vi "AFG3352X.ProcCases.vi"(0 "i ref in":refnum<vi>, 1 "selector":string, 2 "Data":T1, 3 "call cluster":T2={"Object"="", "Selector"="", "CallType"=enum."synchronous", "Async Object"="", "Async Selector"="", "Data Descriptor"="", "Data"=[], "Error #"=0, "Expire"=0}, 5 "error in (no error)":errorcluster) -> (14 "i ref out":refnum<vi>, 17 "answer cluster":T2={"Object"="", "Selector"="", "CallType"=enum."synchronous", "Async Object"="", "Async Selector"="", "Data Descriptor"="", "Data"=[], "Error #"=0, "Expire"=0}, 19 "error out":errorcluster)   [LabVIEW 2014, in "AFG3352X.lvlib"]
doc: "This method is called by a process from within the default case in the event loop. The methods of a class that are linked to events will be called from THIS method. Add your code here."
uses:
  AFG3352X.lvlib
  CS_Core/CSSystem/CoreDefs/CoreDefs.call_type.ctl
  CS_Core/BaseProcess/BaseProcess.descriptor string definition.ctl
  CS_Core/CSSystem/CoreDefs/CoreDefs.rawDataType.ctl
  CS_Core/CSSystem/CoreLib/CoreLib.string 2 byte array.vi
  CS_Core/CSSystem/CoreLib/CoreLib.byte array 2 short.vi
  CS_Core/CSSystem/CoreLib/CoreLib.byte array 2 string.vi
  CS_Core/CSSystem/CoreLib/CoreLib.byte array 2 short array.vi
  CS_Core/CSSystem/CoreLib/CoreLib.byte array 2 int.vi
  CS_Core/CSSystem/CoreLib/CoreLib.byte array 2 double.vi
  CS_Core/CSSystem/CoreLib/CoreLib.byte array 2 double array.vi
  CS_Core/CSSystem/CoreLib/CoreLib.lvlib
  CS_Core/BaseProcess/BaseProcess.lvlib
  CS_Core/CSApplicationBaseClasses/AFGBase/AFGBase.lvlib
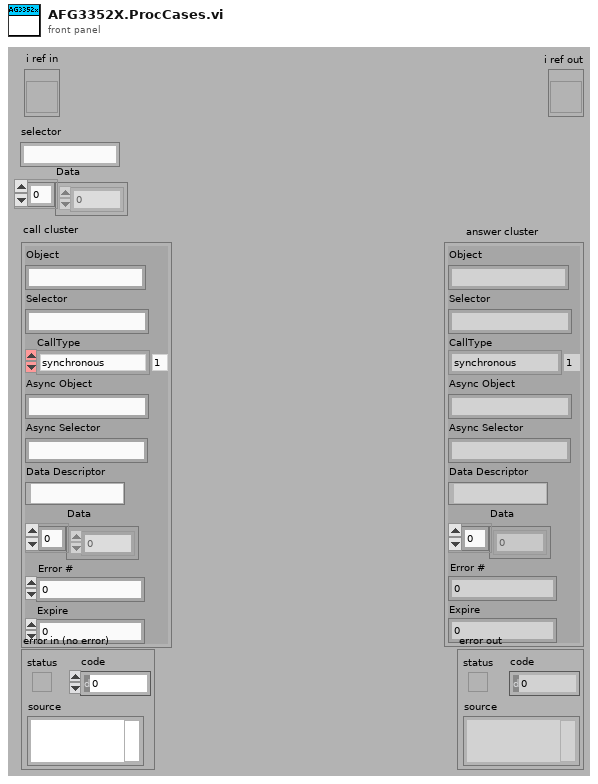
[diagram p1: front panel]
types:
  T1 = typedef "CoreDefs.rawDataType.ctl" = i8[]
  T2 = typedef "CoreDefs.call_type.ctl" = cluster{"Object":string, "Selector":string, "CallType":enum16{"simple", "synchronous", "asynchronous"}, "Async Object":string, "Async Selector":string, "Data Descriptor":T3, "Data":T1, "Error #":i32, "Expire":u32}
  T3 = typedef "BaseProcess.lvlib/BaseProcess.descriptor string definition.ctl" = string
  T4 = typedef "AFG3352X.lvlib/AFG3352X.i attribute.ctl" = cluster{"Act2ndValues":cluster{"frequency":dbl, "amplitude":dbl, "phase":dbl, "DCOffset":dbl, "waveformType":T5, "enableOutput":bool, "trigger":i16[], "serviceIDs":cluster{"frequencyID":i32, "amplitudeID":i32, "phaseID":i32, "DCOffsetID":i32, "waveformTypeID":i32, "enableOutputID":i32, "triggerID":i32}, "waveform":cluster{"data":waveform(dbl), "gain":dbl, "offset":dbl, "repetitionRate":dbl, "sampleRate":dbl}}, "Nom2ndValues":cluster{"frequency":dbl, "amplitude":dbl, "phase":dbl, "DCOffset":dbl, "waveformType":T5, "enableOutput":bool, "trigger":i16[], "serviceIDs":cluster{"frequencyID":i32, "amplitudeID":i32, "phaseID":i32, "DCOffsetID":i32, "waveformTypeID":i32, "enableOutputID":i32, "triggerID":i32}, "waveform":cluster{"data":waveform(dbl), "gain":dbl, "offset":dbl, "repetitionRate":dbl, "sampleRate":dbl}}, "DefaultChannel":i32, "ActAddValues":cluster{"Mode1":u16, "serviceIDs":cluster{"Mode1ID":i32, "Mode2ID":i32, "Burst1ID":i32, "Burst2ID":i32}, "Mode2":u16, "Burst1":i32, "Burst2":i32}, "NomAddValues":cluster{"Mode1":u16, "serviceIDs":cluster{"Mode1ID":i32, "Mode2ID":i32, "Burst1ID":i32, "Burst2ID":i32}, "Mode2 2":u16, "Burst1":i32, "Burst2":i32}, "enableBurstMode":bool}
  T5 = typedef "AFGBase.lvlib/AFGBase.waveformType.ctl" = enum16{"sine", "square", "ramp", "pulse", "noise", "DC", "arbitrary", "triangle", "ramp_up", "ramp_down", "amplitude modulation"}
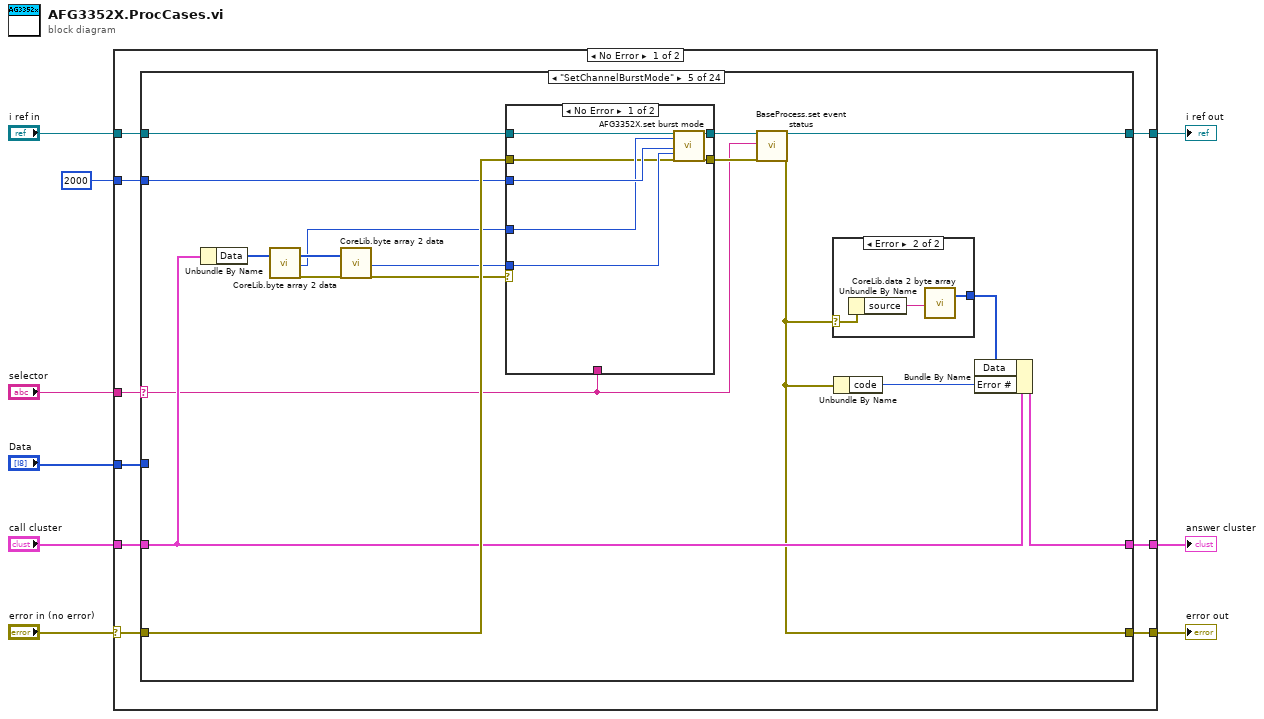
[diagram p0: block diagram]
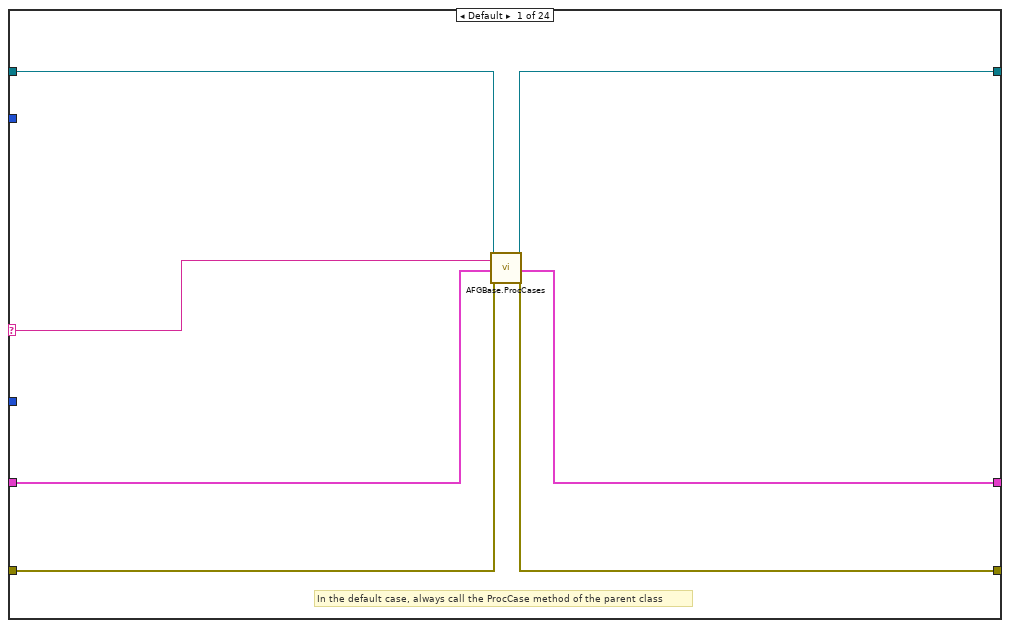
[diagram p2: hidden frame]
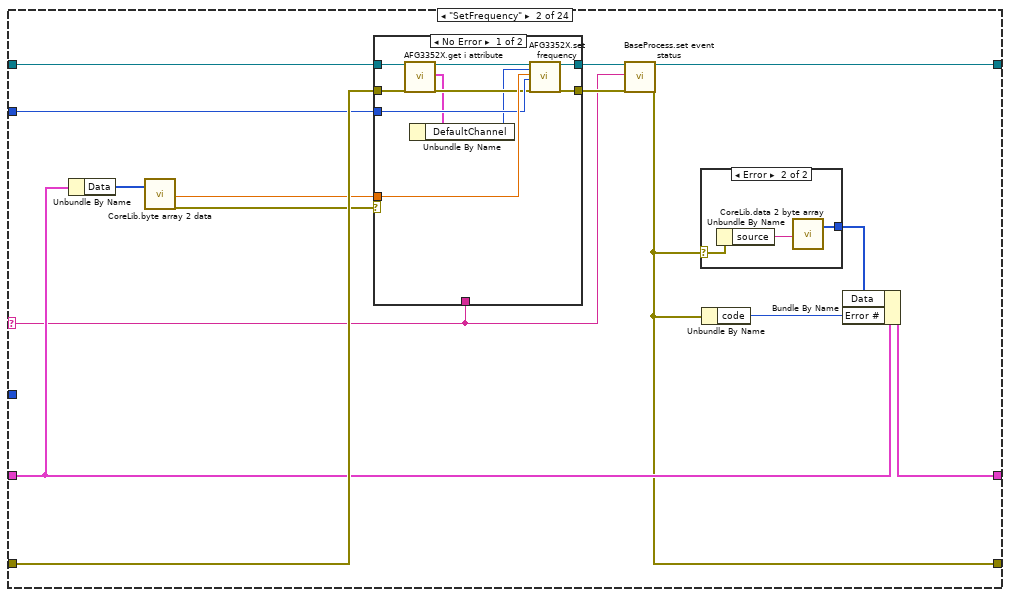
[diagram p3: hidden frame]
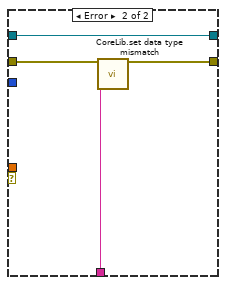
[diagram p5: hidden frame]
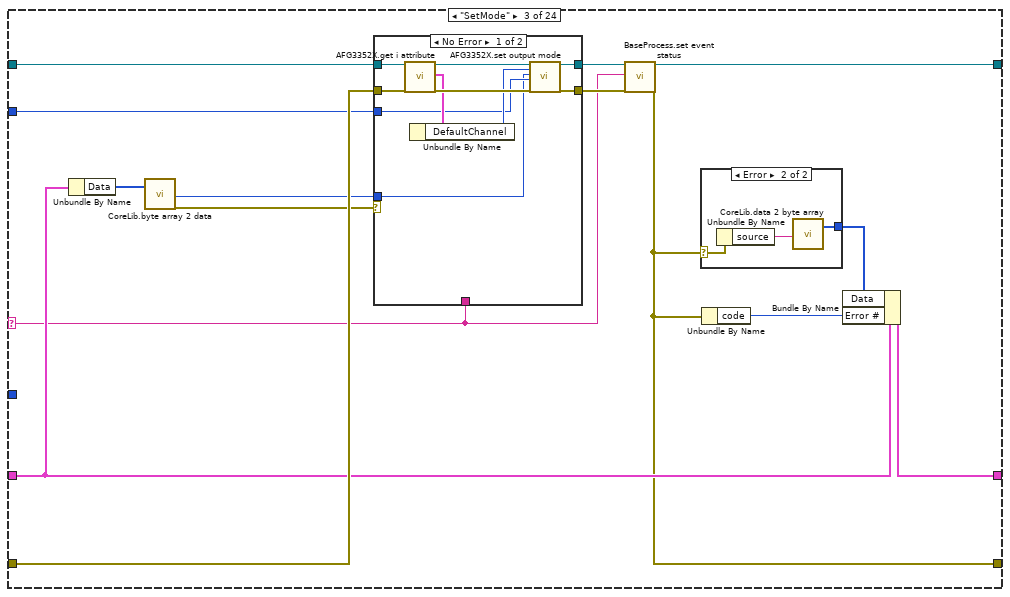
[diagram p6: hidden frame]
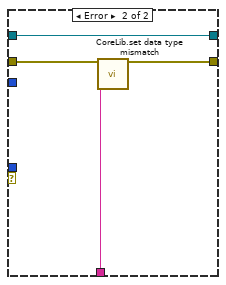
[diagram p8: hidden frame]
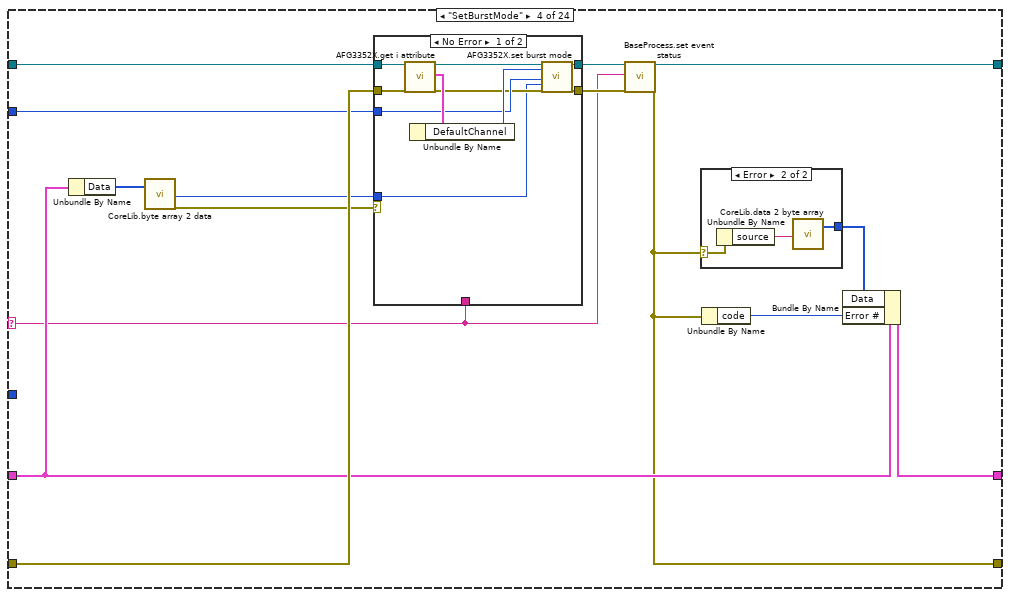
[diagram p9: hidden frame]
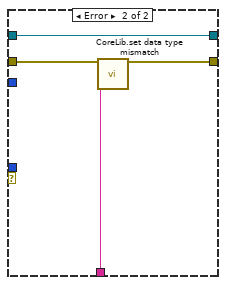
[diagram p11: hidden frame]
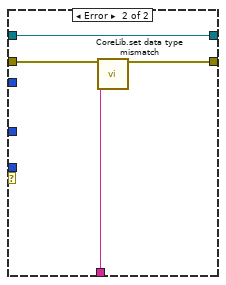
[diagram p13: hidden frame]
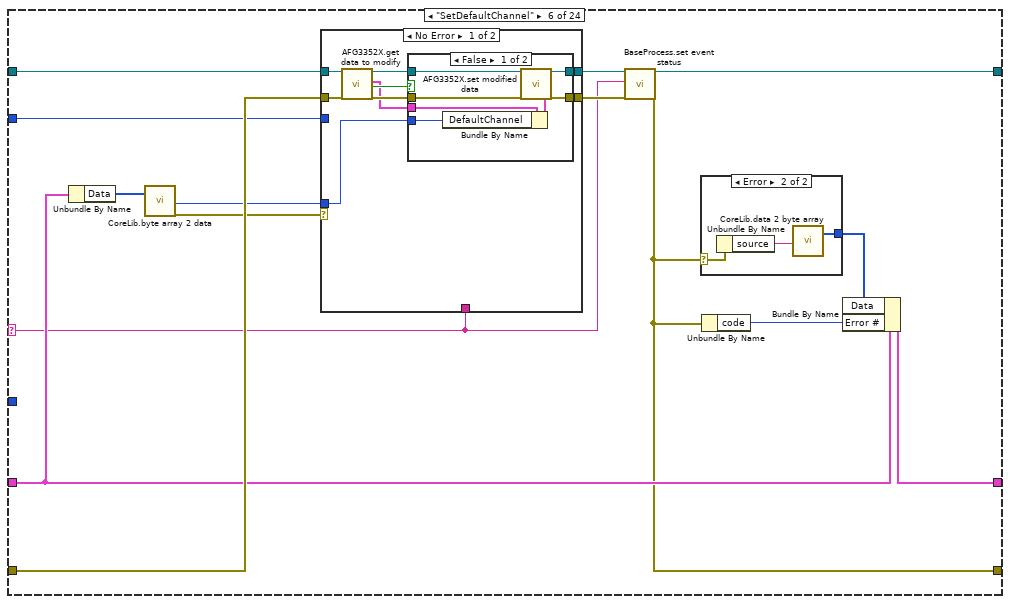
[diagram p14: hidden frame]
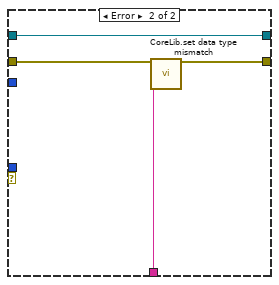
[diagram p17: hidden frame]
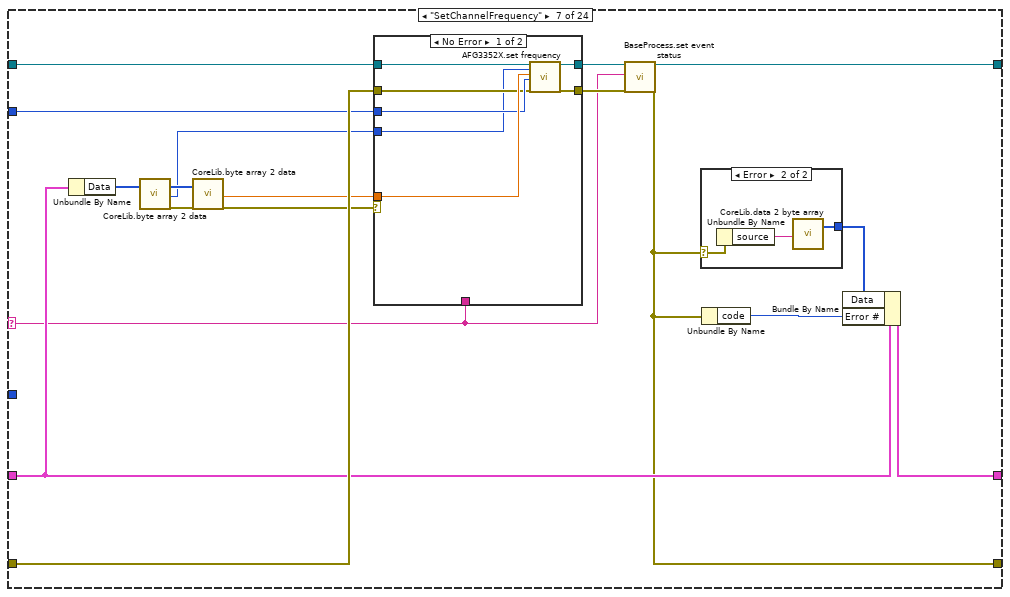
[diagram p18: hidden frame]
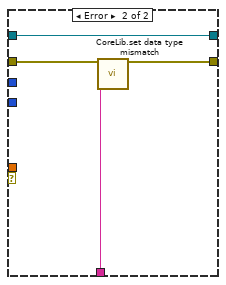
[diagram p20: hidden frame]
diagram:
  n1 = case shown="No Error" "error in (no error)" {
    selector: "error in (no error)" -> [w11 w723]
    tunnel: "selector" -> [w18 _]
    tunnel: [w17 w724] -> w8
    tunnel: "Data" -> [w16 _]
    tunnel: "call cluster" -> [w15 w724]
    tunnel: "i ref in" -> [w14 w725]
    tunnel: [w13 w725] -> w4
    tunnel: [w12 w723] -> w3
    tunnel: 2000 ("ms timeout (10000)") -> [w10 _]
    frame No Error {
      n2 = case shown="\"SetChannelBurstMode\"" w18 {
        selector: w18 -> [w20 w31 w63 w95 w130 w159 w202 w234 w266 w305 w334 w366 w401 w430 w461 w490 w523 w559 w588 w617 w642 w657 w702 w714]
        tunnel: w16 -> [_ _ _ _ _ _ _ _ _ _ _ _ _ _ _ _ _ _ _ _ _ _ _ _]
        tunnel: w14 -> [w19 w40 w72 w104 w139 w168 w211 w243 w275 w313 w343 w375 w410 w439 w470 w499 w532 w568 w597 w626 w651 w665 w698 w712]
        tunnel: [w25 w30 w62 w94 w129 w158 w201 w233 w265 w304 w333 w365 w400 w429 w460 w489 w522 w558 w587 w616 w641 w668 w701 w713] -> w13
        tunnel: w15 -> [w21 w37 w69 w101 w136 w165 w208 w240 w272 w311 w340 w372 w407 w436 w467 w496 w529 w565 w594 w623 w648 w661 w706 w718]
        tunnel: [w22 w36 w68 w100 w135 w164 w207 w239 w271 w310 w339 w371 w406 w435 w466 w495 w528 w564 w593 w622 w647 w673 w705 w717] -> w17
        tunnel: w11 -> [w24 w39 w71 w103 w138 w167 w210 w242 w274 w291 w342 w374 w409 w438 w469 w498 w531 w567 w596 w625 w650 w666 w699 w711]
        tunnel: [w23 w32 w64 w96 w131 w160 w203 w235 w267 w306 w335 w367 w402 w431 w462 w491 w524 w560 w589 w618 w643 w669 w703 w715] -> w12
        tunnel: w10 -> [_ w26 w58 w91 w127 w154 w198 w230 w262 w301 w329 w361 w397 w425 w457 w486 w518 w555 w584 w613 w640 w667 w700 _]
        frame Default {
          # "In the default case, always call the ProcCase method of the parent class"
          n3 = call "AFGBase.ProcCases.vi"("i ref in"=w19, "selector"=w20, "call cluster"=w21, "error in (no error)"=w24) -> ("i ref out"=w25:refnum<vi>, "answer cluster"=w22:T2, "error out"=w23:errorcluster)  [unwired: 13 in]
        }
        frame "SetFrequency" {
          n4 = Unbundle By Name(w37) -> ("Data"=w29:T1)
          n5 = call-poly "CoreLib.byte array 2 data.vi"("byteArray"=w29) -> ("d64"=w28:dbl, "error out"=w27:errorcluster)  [unwired: 16 in, 1 out]
          n6 = case shown="No Error" w27 {
            tunnel: [w53 w57] -> w34
            tunnel: w40 -> [w49 w57]
            tunnel: w39 -> [w46 w56]
            tunnel: [w52 w55] -> w33
            tunnel: w31 -> [_ w54]
            tunnel: w28 -> [w51 _]
            tunnel: w26 -> [w50 _]
            frame No Error {
              n7 = call "AFG3352X.get i attribute.vi"("i ref in"=w49, "error in (no error)"=w46) -> ("i ref out"=w48:refnum<vi>, "i attribute"=w45:T4, "error out"=w47:errorcluster)  [unwired: 15 in]
              n8 = Unbundle By Name(w45) -> ("DefaultChannel"=w44:i32)
              n9 = call "AFG3352X.set frequency.vi"("i ref in"=w48, "Channel (1: 1)"=w44, "frequency [Hz]"=w51, "ms timeout (10000)"=w50, "error in (no error)"=w47) -> ("i ref out"=w53:refnum<vi>, "error out"=w52:errorcluster)  [unwired: 12 in, 1 out]
            }
            frame Error {
              n10 = call "CoreLib.set data type mismatch.vi"("error in (no error)"=w56, "error source"=w54) -> ("error out"=w55:errorcluster)  [unwired: 17 in]
            }
          }
          n11 = call "BaseProcess.set event status.vi"("i ref in"=w34, "EventStatus"=w31, "error in (no error)"=w33) -> ("i ref out"=w30:refnum<vi>, "error out"=w32:errorcluster)  [unwired: 14 in, 1 out]
          n12 = case shown="Error" w32 {
            selector: w32 -> [_ w43]
            tunnel: [_ w42] -> w35
            frame No Error {
            }
            frame Error {
              n13 = Unbundle By Name(w43) -> ("source"=w41:string)
              n14 = call-poly "CoreLib.data 2 byte array.vi"("string"=w41) -> ("byteArray out"=w42:T1)  [unwired: 18 in]
            }
          }
          n15 = Unbundle By Name(w32) -> ("code"=w38:i32)
          n16 = Bundle By Name(cluster=w37, "Data"=w35, "Error #"=w38) -> (w36:T2)
        }
        frame "SetMode" {
          n17 = Unbundle By Name(w69) -> ("Data"=w61:T1)
          n18 = call-poly "CoreLib.byte array 2 data.vi"("byteArray"=w61) -> ("i32"=w60:i32, "error out"=w59:errorcluster)  [unwired: 16 in, 1 out]
          n19 = case shown="No Error" w59 {
            tunnel: [w85 w89] -> w66
            tunnel: w72 -> [w83 w89]
            tunnel: w71 -> [w80 w88]
            tunnel: [w84 w87] -> w65
            tunnel: w63 -> [_ w86]
            tunnel: w60 -> [w76 _]
            tunnel: w58 -> [w77 _]
            frame No Error {
              n20 = call "AFG3352X.get i attribute.vi"("i ref in"=w83, "error in (no error)"=w80) -> ("i ref out"=w82:refnum<vi>, "i attribute"=w79:T4, "error out"=w81:errorcluster)  [unwired: 15 in]
              n21 = Unbundle By Name(w79) -> ("DefaultChannel"=w78:i32)
              n22 = call "AFG3352X.set output mode.vi"("i ref in"=w82, "Channel (1: 1)"=w78, "Output State (0: Normal)"=w76, "ms timeout (10000)"=w77, "error in (no error)"=w81) -> ("i ref out"=w85:refnum<vi>, "error out"=w84:errorcluster)  [unwired: 12 in, 1 out]
            }
            frame Error {
              n23 = call "CoreLib.set data type mismatch.vi"("error in (no error)"=w88, "error source"=w86) -> ("error out"=w87:errorcluster)  [unwired: 17 in]
            }
          }
          n24 = call "BaseProcess.set event status.vi"("i ref in"=w66, "EventStatus"=w63, "error in (no error)"=w65) -> ("i ref out"=w62:refnum<vi>, "error out"=w64:errorcluster)  [unwired: 14 in, 1 out]
          n25 = case shown="Error" w64 {
            selector: w64 -> [_ w75]
            tunnel: [_ w74] -> w67
            frame No Error {
            }
            frame Error {
              n26 = Unbundle By Name(w75) -> ("source"=w73:string)
              n27 = call-poly "CoreLib.data 2 byte array.vi"("string"=w73) -> ("byteArray out"=w74:T1)  [unwired: 18 in]
            }
          }
          n28 = Unbundle By Name(w64) -> ("code"=w70:i32)
          n29 = Bundle By Name(cluster=w69, "Data"=w67, "Error #"=w70) -> (w68:T2)
        }
        frame "SetBurstMode" {
          n30 = Unbundle By Name(w101) -> ("Data"=w93:T1)
          n31 = call-poly "CoreLib.byte array 2 data.vi"("byteArray"=w93) -> ("i32"=w92:i32, "error out"=w90:errorcluster)  [unwired: 16 in, 1 out]
          n32 = case shown="No Error" w90 {
            tunnel: [w114 w121] -> w98
            tunnel: w104 -> [w117 w121]
            tunnel: w103 -> [w116 w120]
            tunnel: [w113 w119] -> w97
            tunnel: w95 -> [_ w118]
            tunnel: w92 -> [w108 _]
            tunnel: w91 -> [w110 _]
            frame No Error {
              n33 = call "AFG3352X.get i attribute.vi"("i ref in"=w117, "error in (no error)"=w116) -> ("i ref out"=w112:refnum<vi>, "i attribute"=w115:T4, "error out"=w109:errorcluster)  [unwired: 15 in]
              n34 = Unbundle By Name(w115) -> ("DefaultChannel"=w111:i32)
              n35 = call "AFG3352X.set burst mode.vi"("i ref in"=w112, "Channel (1: 1)"=w111, "ms timeout (10000)"=w110, "Burst Mode \n(0: Triggered)"=w108, "error in (no error)"=w109) -> ("i ref out"=w114:refnum<vi>, "error out"=w113:errorcluster)  [unwired: 12 in, 1 out]
            }
            frame Error {
              n36 = call "CoreLib.set data type mismatch.vi"("error in (no error)"=w120, "error source"=w118) -> ("error out"=w119:errorcluster)  [unwired: 17 in]
            }
          }
          n37 = call "BaseProcess.set event status.vi"("i ref in"=w98, "EventStatus"=w95, "error in (no error)"=w97) -> ("i ref out"=w94:refnum<vi>, "error out"=w96:errorcluster)  [unwired: 14 in, 1 out]
          n38 = case shown="Error" w96 {
            selector: w96 -> [_ w107]
            tunnel: [_ w106] -> w99
            frame No Error {
            }
            frame Error {
              n39 = Unbundle By Name(w107) -> ("source"=w105:string)
              n40 = call-poly "CoreLib.data 2 byte array.vi"("string"=w105) -> ("byteArray out"=w106:T1)  [unwired: 18 in]
            }
          }
          n41 = Unbundle By Name(w96) -> ("code"=w102:i32)
          n42 = Bundle By Name(cluster=w101, "Data"=w99, "Error #"=w102) -> (w100:T2)
        }
        frame "SetChannelBurstMode" {
          n43 = Unbundle By Name(w136) -> ("Data"=w123:T1)
          n44 = call-poly "CoreLib.byte array 2 data.vi"("byteArray"=w123) -> ("byteArray out"=w124:T1, "i32"=w122:i32, "error out"=w125:errorcluster)  [unwired: 16 in]
          n45 = call-poly "CoreLib.byte array 2 data.vi"("byteArray"=w124, "error in (no error)"=w125) -> ("i32"=w128:i32, "error out"=w126:errorcluster)  [unwired: 15 in, 1 out]
          n46 = case shown="No Error" w126 {
            tunnel: [w149 w153] -> w133
            tunnel: w139 -> [w144 w153]
            tunnel: w138 -> [w143 w152]
            tunnel: [w148 w151] -> w132
            tunnel: w130 -> [_ w150]
            tunnel: w128 -> [w146 _]
            tunnel: w127 -> [w147 _]
            tunnel: w122 -> [w145 _]
            frame No Error {
              n47 = call "AFG3352X.set burst mode.vi"("i ref in"=w144, "Channel (1: 1)"=w145, "ms timeout (10000)"=w147, "Burst Mode \n(0: Triggered)"=w146, "error in (no error)"=w143) -> ("i ref out"=w149:refnum<vi>, "error out"=w148:errorcluster)  [unwired: 12 in, 1 out]
            }
            frame Error {
              n48 = call "CoreLib.set data type mismatch.vi"("error in (no error)"=w152, "error source"=w150) -> ("error out"=w151:errorcluster)  [unwired: 17 in]
            }
          }
          n49 = call "BaseProcess.set event status.vi"("i ref in"=w133, "EventStatus"=w130, "error in (no error)"=w132) -> ("i ref out"=w129:refnum<vi>, "error out"=w131:errorcluster)  [unwired: 14 in, 1 out]
          n50 = case shown="Error" w131 {
            selector: w131 -> [_ w142]
            tunnel: [_ w141] -> w134
            frame No Error {
            }
            frame Error {
              n51 = Unbundle By Name(w142) -> ("source"=w140:string)
              n52 = call-poly "CoreLib.data 2 byte array.vi"("string"=w140) -> ("byteArray out"=w141:T1)  [unwired: 18 in]
            }
          }
          n53 = Unbundle By Name(w131) -> ("code"=w137:i32)
          n54 = Bundle By Name(cluster=w136, "Data"=w134, "Error #"=w137) -> (w135:T2)
        }
        frame "SetDefaultChannel" {
          n55 = Unbundle By Name(w165) -> ("Data"=w157:T1)
          n56 = call-poly "CoreLib.byte array 2 data.vi"("byteArray"=w157) -> ("i32"=w156:i32, "error out"=w155:errorcluster)  [unwired: 16 in, 1 out]
          n57 = case shown="No Error" w155 {
            tunnel: [w176 w193] -> w162
            tunnel: w168 -> [w180 w193]
            tunnel: w167 -> [w179 w192]
            tunnel: [w175 w191] -> w161
            tunnel: w159 -> [_ w190]
            tunnel: w156 -> [w172 _]
            tunnel: w154 -> [_ _]
            frame No Error {
              n58 = call "AFG3352X.get data to modify.vi"("i ref in"=w180, "error in (no error)"=w179) -> ("i ref out"=w178:refnum<vi>, "i attribute"=w173:T4, "timed out"=w174:bool, "error out"=w177:errorcluster)  [unwired: 14 in]
              n59 = case shown="False" w174 {
                tunnel: w178 -> [w187 w189]
                tunnel: w177 -> [w186 w188]
                tunnel: [w185 w189] -> w176
                tunnel: [w184 w188] -> w175
                tunnel: w173 -> [w183 _]
                tunnel: w172 -> [w181 _]
                frame False {
                  n60 = Bundle By Name(cluster=w183, "DefaultChannel"=w181) -> (w182:T4)
                  n61 = call "AFG3352X.set modified data.vi"("i ref in"=w187, "i attribute"=w182, "error in (no error)"=w186) -> ("i ref out"=w185:refnum<vi>, "error out"=w184:errorcluster)  [unwired: 15 in]
                }
                frame True {
                }
              }
            }
            frame Error {
              n62 = call "CoreLib.set data type mismatch.vi"("error in (no error)"=w192, "error source"=w190) -> ("error out"=w191:errorcluster)  [unwired: 17 in]
            }
          }
          n63 = call "BaseProcess.set event status.vi"("i ref in"=w162, "EventStatus"=w159, "error in (no error)"=w161) -> ("i ref out"=w158:refnum<vi>, "error out"=w160:errorcluster)  [unwired: 14 in, 1 out]
          n64 = case shown="Error" w160 {
            selector: w160 -> [_ w171]
            tunnel: [_ w170] -> w163
            frame No Error {
            }
            frame Error {
              n65 = Unbundle By Name(w171) -> ("source"=w169:string)
              n66 = call-poly "CoreLib.data 2 byte array.vi"("string"=w169) -> ("byteArray out"=w170:T1)  [unwired: 18 in]
            }
          }
          n67 = Unbundle By Name(w160) -> ("code"=w166:i32)
          n68 = Bundle By Name(cluster=w165, "Data"=w163, "Error #"=w166) -> (w164:T2)
        }
        frame "SetChannelFrequency" {
          n69 = Unbundle By Name(w208) -> ("Data"=w195:T1)
          n70 = call-poly "CoreLib.byte array 2 data.vi"("byteArray"=w195) -> ("byteArray out"=w197:T1, "i32"=w194:i32, "error out"=w196:errorcluster)  [unwired: 16 in]
          n71 = call-poly "CoreLib.byte array 2 data.vi"("byteArray"=w197, "error in (no error)"=w196) -> ("d64"=w200:dbl, "error out"=w199:errorcluster)  [unwired: 15 in, 1 out]
          n72 = case shown="No Error" w199 {
            tunnel: [w221 w225] -> w205
            tunnel: w211 -> [w216 w225]
            tunnel: w210 -> [w217 w224]
            tunnel: [w220 w223] -> w204
            tunnel: w202 -> [_ w222]
            tunnel: w200 -> [w219 _]
            tunnel: w198 -> [w218 _]
            tunnel: w194 -> [w215 _]
            frame No Error {
              n73 = call "AFG3352X.set frequency.vi"("i ref in"=w216, "Channel (1: 1)"=w215, "frequency [Hz]"=w219, "ms timeout (10000)"=w218, "error in (no error)"=w217) -> ("i ref out"=w221:refnum<vi>, "error out"=w220:errorcluster)  [unwired: 12 in, 1 out]
            }
            frame Error {
              n74 = call "CoreLib.set data type mismatch.vi"("error in (no error)"=w224, "error source"=w222) -> ("error out"=w223:errorcluster)  [unwired: 17 in]
            }
          }
          n75 = call "BaseProcess.set event status.vi"("i ref in"=w205, "EventStatus"=w202, "error in (no error)"=w204) -> ("i ref out"=w201:refnum<vi>, "error out"=w203:errorcluster)  [unwired: 14 in, 1 out]
          n76 = case shown="Error" w203 {
            selector: w203 -> [_ w214]
            tunnel: [_ w213] -> w206
            frame No Error {
            }
            frame Error {
              n77 = Unbundle By Name(w214) -> ("source"=w212:string)
              n78 = call-poly "CoreLib.data 2 byte array.vi"("string"=w212) -> ("byteArray out"=w213:T1)  [unwired: 18 in]
            }
          }
          n79 = Unbundle By Name(w203) -> ("code"=w209:i32)
          n80 = Bundle By Name(cluster=w208, "Data"=w206, "Error #"=w209) -> (w207:T2)
        }
        frame "SetChannelMode" {
          n81 = Unbundle By Name(w240) -> ("Data"=w227:T1)
          n82 = call-poly "CoreLib.byte array 2 data.vi"("byteArray"=w227) -> ("byteArray out"=w229:T1, "i32"=w226:i32, "error out"=w228:errorcluster)  [unwired: 16 in]
          n83 = call-poly "CoreLib.byte array 2 data.vi"("byteArray"=w229, "error in (no error)"=w228) -> ("i32"=w232:i32, "error out"=w231:errorcluster)  [unwired: 15 in, 1 out]
          n84 = case shown="No Error" w231 {
            tunnel: [w253 w257] -> w237
            tunnel: w243 -> [w248 w257]
            tunnel: w242 -> [w249 w256]
            tunnel: [w252 w255] -> w236
            tunnel: w234 -> [_ w254]
            tunnel: w232 -> [w251 _]
            tunnel: w230 -> [w250 _]
            tunnel: w226 -> [w247 _]
            frame No Error {
              n85 = call "AFG3352X.set output mode.vi"("i ref in"=w248, "Channel (1: 1)"=w247, "Output State (0: Normal)"=w251, "ms timeout (10000)"=w250, "error in (no error)"=w249) -> ("i ref out"=w253:refnum<vi>, "error out"=w252:errorcluster)  [unwired: 12 in, 1 out]
            }
            frame Error {
              n86 = call "CoreLib.set data type mismatch.vi"("error in (no error)"=w256, "error source"=w254) -> ("error out"=w255:errorcluster)  [unwired: 17 in]
            }
          }
          n87 = call "BaseProcess.set event status.vi"("i ref in"=w237, "EventStatus"=w234, "error in (no error)"=w236) -> ("i ref out"=w233:refnum<vi>, "error out"=w235:errorcluster)  [unwired: 14 in, 1 out]
          n88 = case shown="Error" w235 {
            selector: w235 -> [_ w246]
            tunnel: [_ w245] -> w238
            frame No Error {
            }
            frame Error {
              n89 = Unbundle By Name(w246) -> ("source"=w244:string)
              n90 = call-poly "CoreLib.data 2 byte array.vi"("string"=w244) -> ("byteArray out"=w245:T1)  [unwired: 18 in]
            }
          }
          n91 = Unbundle By Name(w235) -> ("code"=w241:i32)
          n92 = Bundle By Name(cluster=w240, "Data"=w238, "Error #"=w241) -> (w239:T2)
        }
        frame "SetChannelPhase" {
          n93 = Unbundle By Name(w272) -> ("Data"=w259:T1)
          n94 = call-poly "CoreLib.byte array 2 data.vi"("byteArray"=w259) -> ("byteArray out"=w261:T1, "i32"=w258:i32, "error out"=w260:errorcluster)  [unwired: 16 in]
          n95 = call-poly "CoreLib.byte array 2 data.vi"("byteArray"=w261, "error in (no error)"=w260) -> ("d64"=w264:dbl, "error out"=w263:errorcluster)  [unwired: 15 in, 1 out]
          n96 = case shown="No Error" w263 {
            tunnel: [w285 w289] -> w269
            tunnel: w275 -> [w280 w289]
            tunnel: w274 -> [w281 w288]
            tunnel: [w284 w287] -> w268
            tunnel: w266 -> [_ w286]
            tunnel: w264 -> [w283 _]
            tunnel: w262 -> [w282 _]
            tunnel: w258 -> [w279 _]
            frame No Error {
              n97 = call "AFG3352X.set phase.vi"("i ref in"=w280, "Channel (1: 1)"=w279, "Phase Angle (0 Degree)"=w283, "ms timeout (10000)"=w282, "error in (no error)"=w281) -> ("i ref out"=w285:refnum<vi>, "error out"=w284:errorcluster)  [unwired: 12 in, 1 out]
            }
            frame Error {
              n98 = call "CoreLib.set data type mismatch.vi"("error in (no error)"=w288, "error source"=w286) -> ("error out"=w287:errorcluster)  [unwired: 17 in]
            }
          }
          n99 = call "BaseProcess.set event status.vi"("i ref in"=w269, "EventStatus"=w266, "error in (no error)"=w268) -> ("i ref out"=w265:refnum<vi>, "error out"=w267:errorcluster)  [unwired: 14 in, 1 out]
          n100 = case shown="Error" w267 {
            selector: w267 -> [_ w278]
            tunnel: [_ w277] -> w270
            frame No Error {
            }
            frame Error {
              n101 = Unbundle By Name(w278) -> ("source"=w276:string)
              n102 = call-poly "CoreLib.data 2 byte array.vi"("string"=w276) -> ("byteArray out"=w277:T1)  [unwired: 18 in]
            }
          }
          n103 = Unbundle By Name(w267) -> ("code"=w273:i32)
          n104 = Bundle By Name(cluster=w272, "Data"=w270, "Error #"=w273) -> (w271:T2)
        }
        frame "SetSWIFT" {
          n105 = Unbundle By Name(w311) -> ("Data"=w303:T1)
          n106 = call-poly "CoreLib.byte array 2 data.vi"("byteArray"=w303) -> ("byteArray out"=w300:T1, "d64"=w302:dbl, "error out"=w299:errorcluster)  [unwired: 16 in]
          n107 = call-poly "CoreLib.byte array 2 data.vi"("byteArray"=w300, "error in (no error)"=w299) -> ("byteArray out"=w297:T1, "d64"=w298:dbl, "error out"=w296:errorcluster)  [unwired: 15 in]
          n108 = call-poly "CoreLib.byte array 2 data.vi"("byteArray"=w297, "error in (no error)"=w296) -> ("byteArray out"=w293:T1, "d64"=w295:dbl, "error out"=w294:errorcluster)  [unwired: 15 in]
          n109 = call-poly "CoreLib.byte array 2 data.vi"("byteArray"=w293, "error in (no error)"=w294) -> ("[d64]"=w292:dbl[], "error out"=w290:errorcluster)  [unwired: 15 in, 1 out]
          n110 = case shown="No Error" w290 {
            tunnel: [w323 w328] -> w308
            tunnel: w313 -> [w324 w328]
            tunnel: w291 -> [w322 w327]
            tunnel: [w321 w326] -> w307
            tunnel: w305 -> [_ w325]
            tunnel: w302 -> [w320 _]
            tunnel: w301 -> [_ _]
            tunnel: w298 -> [w319 _]
            tunnel: w295 -> [w318 _]
            tunnel: w292 -> [w317 _]
            frame No Error {
              n111 = call "AFG3352X.set SWIFT.vi"("i ref in"=w324, "Amplitude (0.1 Vpp)"=w320, "Offset (0 V)"=w319, "Sample Rate (40000 Sa/s)"=w318, "Apodized SWIFT"=w317, "error in (no error)"=w322) -> ("i ref out"=w323:refnum<vi>, "error out"=w321:errorcluster)  [unwired: 12 in]
            }
            frame Error {
              n112 = call "CoreLib.set data type mismatch.vi"("error in (no error)"=w327, "error source"=w325) -> ("error out"=w326:errorcluster)  [unwired: 17 in]
            }
          }
          n113 = call "BaseProcess.set event status.vi"("i ref in"=w308, "EventStatus"=w305, "error in (no error)"=w307) -> ("i ref out"=w304:refnum<vi>, "error out"=w306:errorcluster)  [unwired: 14 in, 1 out]
          n114 = case shown="Error" w306 {
            selector: w306 -> [_ w316]
            tunnel: [_ w315] -> w309
            frame No Error {
            }
            frame Error {
              n115 = Unbundle By Name(w316) -> ("source"=w314:string)
              n116 = call-poly "CoreLib.data 2 byte array.vi"("string"=w314) -> ("byteArray out"=w315:T1)  [unwired: 18 in]
            }
          }
          n117 = Unbundle By Name(w306) -> ("code"=w312:i32)
          n118 = Bundle By Name(cluster=w311, "Data"=w309, "Error #"=w312) -> (w310:T2)
        }
        frame "SetAmplitude" {
          n119 = Unbundle By Name(w340) -> ("Data"=w332:T1)
          n120 = call-poly "CoreLib.byte array 2 data.vi"("byteArray"=w332) -> ("d64"=w331:dbl, "error out"=w330:errorcluster)  [unwired: 16 in, 1 out]
          n121 = case shown="No Error" w330 {
            tunnel: [w356 w360] -> w337
            tunnel: w343 -> [w349 w360]
            tunnel: w342 -> [w352 w359]
            tunnel: [w355 w358] -> w336
            tunnel: w334 -> [_ w357]
            tunnel: w331 -> [w354 _]
            tunnel: w329 -> [w353 _]
            frame No Error {
              n122 = call "AFG3352X.get i attribute.vi"("i ref in"=w349, "error in (no error)"=w352) -> ("i ref out"=w350:refnum<vi>, "i attribute"=w348:T4, "error out"=w351:errorcluster)  [unwired: 15 in]
              n123 = Unbundle By Name(w348) -> ("DefaultChannel"=w347:i32)
              n124 = call "AFG3352X.set amplitude.vi"("i ref in"=w350, "Channel (1: 1)"=w347, "amplitude [V]"=w354, "ms timeout (10000)"=w353, "error in (no error)"=w351) -> ("i ref out"=w356:refnum<vi>, "error out"=w355:errorcluster)  [unwired: 12 in, 1 out]
            }
            frame Error {
              n125 = call "CoreLib.set data type mismatch.vi"("error in (no error)"=w359, "error source"=w357) -> ("error out"=w358:errorcluster)  [unwired: 17 in]
            }
          }
          n126 = call "BaseProcess.set event status.vi"("i ref in"=w337, "EventStatus"=w334, "error in (no error)"=w336) -> ("i ref out"=w333:refnum<vi>, "error out"=w335:errorcluster)  [unwired: 14 in, 1 out]
          n127 = case shown="Error" w335 {
            selector: w335 -> [_ w346]
            tunnel: [_ w345] -> w338
            frame No Error {
            }
            frame Error {
              n128 = Unbundle By Name(w346) -> ("source"=w344:string)
              n129 = call-poly "CoreLib.data 2 byte array.vi"("string"=w344) -> ("byteArray out"=w345:T1)  [unwired: 18 in]
            }
          }
          n130 = Unbundle By Name(w335) -> ("code"=w341:i32)
          n131 = Bundle By Name(cluster=w340, "Data"=w338, "Error #"=w341) -> (w339:T2)
        }
        frame "SetPhase" {
          n132 = Unbundle By Name(w372) -> ("Data"=w364:T1)
          n133 = call-poly "CoreLib.byte array 2 data.vi"("byteArray"=w364) -> ("d64"=w363:dbl, "error out"=w362:errorcluster)  [unwired: 16 in, 1 out]
          n134 = case shown="No Error" w362 {
            tunnel: [w388 w392] -> w369
            tunnel: w375 -> [w381 w392]
            tunnel: w374 -> [w384 w391]
            tunnel: [w387 w390] -> w368
            tunnel: w366 -> [_ w389]
            tunnel: w363 -> [w386 _]
            tunnel: w361 -> [w385 _]
            frame No Error {
              n135 = call "AFG3352X.get i attribute.vi"("i ref in"=w381, "error in (no error)"=w384) -> ("i ref out"=w382:refnum<vi>, "i attribute"=w380:T4, "error out"=w383:errorcluster)  [unwired: 15 in]
              n136 = Unbundle By Name(w380) -> ("DefaultChannel"=w379:i32)
              n137 = call "AFG3352X.set phase.vi"("i ref in"=w382, "Channel (1: 1)"=w379, "Phase Angle (0 Degree)"=w386, "ms timeout (10000)"=w385, "error in (no error)"=w383) -> ("i ref out"=w388:refnum<vi>, "error out"=w387:errorcluster)  [unwired: 12 in, 1 out]
            }
            frame Error {
              n138 = call "CoreLib.set data type mismatch.vi"("error in (no error)"=w391, "error source"=w389) -> ("error out"=w390:errorcluster)  [unwired: 17 in]
            }
          }
          n139 = call "BaseProcess.set event status.vi"("i ref in"=w369, "EventStatus"=w366, "error in (no error)"=w368) -> ("i ref out"=w365:refnum<vi>, "error out"=w367:errorcluster)  [unwired: 14 in, 1 out]
          n140 = case shown="Error" w367 {
            selector: w367 -> [_ w378]
            tunnel: [_ w377] -> w370
            frame No Error {
            }
            frame Error {
              n141 = Unbundle By Name(w378) -> ("source"=w376:string)
              n142 = call-poly "CoreLib.data 2 byte array.vi"("string"=w376) -> ("byteArray out"=w377:T1)  [unwired: 18 in]
            }
          }
          n143 = Unbundle By Name(w367) -> ("code"=w373:i32)
          n144 = Bundle By Name(cluster=w372, "Data"=w370, "Error #"=w373) -> (w371:T2)
        }
        frame "SetChannelAmplitude" {
          n145 = Unbundle By Name(w407) -> ("Data"=w394:T1)
          n146 = call-poly "CoreLib.byte array 2 data.vi"("byteArray"=w394) -> ("byteArray out"=w396:T1, "i32"=w393:i32, "error out"=w395:errorcluster)  [unwired: 16 in]
          n147 = call-poly "CoreLib.byte array 2 data.vi"("byteArray"=w396, "error in (no error)"=w395) -> ("d64"=w399:dbl, "error out"=w398:errorcluster)  [unwired: 15 in, 1 out]
          n148 = case shown="No Error" w398 {
            tunnel: [w420 w424] -> w404
            tunnel: w410 -> [w415 w424]
            tunnel: w409 -> [w416 w423]
            tunnel: [w419 w422] -> w403
            tunnel: w401 -> [_ w421]
            tunnel: w399 -> [w418 _]
            tunnel: w397 -> [w417 _]
            tunnel: w393 -> [w414 _]
            frame No Error {
              n149 = call "AFG3352X.set amplitude.vi"("i ref in"=w415, "Channel (1: 1)"=w414, "amplitude [V]"=w418, "ms timeout (10000)"=w417, "error in (no error)"=w416) -> ("i ref out"=w420:refnum<vi>, "error out"=w419:errorcluster)  [unwired: 12 in, 1 out]
            }
            frame Error {
              n150 = call "CoreLib.set data type mismatch.vi"("error in (no error)"=w423, "error source"=w421) -> ("error out"=w422:errorcluster)  [unwired: 17 in]
            }
          }
          n151 = call "BaseProcess.set event status.vi"("i ref in"=w404, "EventStatus"=w401, "error in (no error)"=w403) -> ("i ref out"=w400:refnum<vi>, "error out"=w402:errorcluster)  [unwired: 14 in, 1 out]
          n152 = case shown="Error" w402 {
            selector: w402 -> [_ w413]
            tunnel: [_ w412] -> w405
            frame No Error {
            }
            frame Error {
              n153 = Unbundle By Name(w413) -> ("source"=w411:string)
              n154 = call-poly "CoreLib.data 2 byte array.vi"("string"=w411) -> ("byteArray out"=w412:T1)  [unwired: 18 in]
            }
          }
          n155 = Unbundle By Name(w402) -> ("code"=w408:i32)
          n156 = Bundle By Name(cluster=w407, "Data"=w405, "Error #"=w408) -> (w406:T2)
        }
        frame "SetGauss" {
          n157 = Unbundle By Name(w436) -> ("Data"=w428:T1)
          n158 = call-poly "CoreLib.byte array 2 data.vi"("byteArray"=w428) -> ("d64"=w427:dbl, "error out"=w426:errorcluster)  [unwired: 16 in, 1 out]
          n159 = case shown="No Error" w426 {
            tunnel: [w447 w452] -> w433
            tunnel: w439 -> [w448 w452]
            tunnel: w438 -> [w445 w451]
            tunnel: [w446 w450] -> w432
            tunnel: w430 -> [_ w449]
            tunnel: w427 -> [w444 _]
            tunnel: w425 -> [w443 _]
            frame No Error {
              n160 = call "AFG3352X.set Gauss.vi"("i ref in"=w448, "Length [us]"=w444, "ms timeout (10000)"=w443, "error in (no error)"=w445) -> ("i ref out"=w447:refnum<vi>, "error out"=w446:errorcluster)  [unwired: 13 in, 1 out]
            }
            frame Error {
              n161 = call "CoreLib.set data type mismatch.vi"("error in (no error)"=w451, "error source"=w449) -> ("error out"=w450:errorcluster)  [unwired: 17 in]
            }
          }
          n162 = call "BaseProcess.set event status.vi"("i ref in"=w433, "EventStatus"=w430, "error in (no error)"=w432) -> ("i ref out"=w429:refnum<vi>, "error out"=w431:errorcluster)  [unwired: 14 in, 1 out]
          n163 = case shown="Error" w431 {
            selector: w431 -> [_ w442]
            tunnel: [_ w441] -> w434
            frame No Error {
            }
            frame Error {
              n164 = Unbundle By Name(w442) -> ("source"=w440:string)
              n165 = call-poly "CoreLib.data 2 byte array.vi"("string"=w440) -> ("byteArray out"=w441:T1)  [unwired: 18 in]
            }
          }
          n166 = Unbundle By Name(w431) -> ("code"=w437:i32)
          n167 = Bundle By Name(cluster=w436, "Data"=w434, "Error #"=w437) -> (w435:T2)
        }
        frame "SetChannelDCOffset" {
          n168 = Unbundle By Name(w467) -> ("Data"=w454:T1)
          n169 = call-poly "CoreLib.byte array 2 data.vi"("byteArray"=w454) -> ("byteArray out"=w456:T1, "i32"=w453:i32, "error out"=w455:errorcluster)  [unwired: 16 in]
          n170 = call-poly "CoreLib.byte array 2 data.vi"("byteArray"=w456, "error in (no error)"=w455) -> ("d64"=w459:dbl, "error out"=w458:errorcluster)  [unwired: 15 in, 1 out]
          n171 = case shown="No Error" w458 {
            tunnel: [w479 w484] -> w464
            tunnel: w470 -> [w480 w484]
            tunnel: w469 -> [w477 w483]
            tunnel: [w478 w482] -> w463
            tunnel: w461 -> [_ w481]
            tunnel: w459 -> [w476 _]
            tunnel: w457 -> [w475 _]
            tunnel: w453 -> [w474 _]
            frame No Error {
              n172 = call "AFG3352X.set DC offset.vi"("i ref in"=w480, "Channel (1: 1)"=w474, "DCOffset [V]"=w476, "ms timeout (10000)"=w475, "error in (no error)"=w477) -> ("i ref out"=w479:refnum<vi>, "error out"=w478:errorcluster)  [unwired: 12 in, 1 out]
            }
            frame Error {
              n173 = call "CoreLib.set data type mismatch.vi"("error in (no error)"=w483, "error source"=w481) -> ("error out"=w482:errorcluster)  [unwired: 17 in]
            }
          }
          n174 = call "BaseProcess.set event status.vi"("i ref in"=w464, "EventStatus"=w461, "error in (no error)"=w463) -> ("i ref out"=w460:refnum<vi>, "error out"=w462:errorcluster)  [unwired: 14 in, 1 out]
          n175 = case shown="Error" w462 {
            selector: w462 -> [_ w473]
            tunnel: [_ w472] -> w465
            frame No Error {
            }
            frame Error {
              n176 = Unbundle By Name(w473) -> ("source"=w471:string)
              n177 = call-poly "CoreLib.data 2 byte array.vi"("string"=w471) -> ("byteArray out"=w472:T1)  [unwired: 18 in]
            }
          }
          n178 = Unbundle By Name(w462) -> ("code"=w468:i32)
          n179 = Bundle By Name(cluster=w467, "Data"=w465, "Error #"=w468) -> (w466:T2)
        }
        frame "SetDCOffset" {
          n180 = Unbundle By Name(w496) -> ("Data"=w485:T1)
          n181 = call-poly "CoreLib.byte array 2 data.vi"("byteArray"=w485) -> ("d64"=w488:dbl, "error out"=w487:errorcluster)  [unwired: 16 in, 1 out]
          n182 = case shown="No Error" w487 {
            tunnel: [w512 w516] -> w493
            tunnel: w499 -> [w506 w516]
            tunnel: w498 -> [w508 w515]
            tunnel: [w511 w514] -> w492
            tunnel: w490 -> [_ w513]
            tunnel: w488 -> [w510 _]
            tunnel: w486 -> [w509 _]
            frame No Error {
              n183 = call "AFG3352X.get i attribute.vi"("i ref in"=w506, "error in (no error)"=w508) -> ("i ref out"=w505:refnum<vi>, "i attribute"=w504:T4, "error out"=w507:errorcluster)  [unwired: 15 in]
              n184 = Unbundle By Name(w504) -> ("DefaultChannel"=w503:i32)
              n185 = call "AFG3352X.set DC offset.vi"("i ref in"=w505, "Channel (1: 1)"=w503, "DCOffset [V]"=w510, "ms timeout (10000)"=w509, "error in (no error)"=w507) -> ("i ref out"=w512:refnum<vi>, "error out"=w511:errorcluster)  [unwired: 12 in, 1 out]
            }
            frame Error {
              n186 = call "CoreLib.set data type mismatch.vi"("error in (no error)"=w515, "error source"=w513) -> ("error out"=w514:errorcluster)  [unwired: 17 in]
            }
          }
          n187 = call "BaseProcess.set event status.vi"("i ref in"=w493, "EventStatus"=w490, "error in (no error)"=w492) -> ("i ref out"=w489:refnum<vi>, "error out"=w491:errorcluster)  [unwired: 14 in, 1 out]
          n188 = case shown="Error" w491 {
            selector: w491 -> [_ w502]
            tunnel: [_ w501] -> w494
            frame No Error {
            }
            frame Error {
              n189 = Unbundle By Name(w502) -> ("source"=w500:string)
              n190 = call-poly "CoreLib.data 2 byte array.vi"("string"=w500) -> ("byteArray out"=w501:T1)  [unwired: 18 in]
            }
          }
          n191 = Unbundle By Name(w491) -> ("code"=w497:i32)
          n192 = Bundle By Name(cluster=w496, "Data"=w494, "Error #"=w497) -> (w495:T2)
        }
        frame "SetOutputEnabled" {
          n193 = Unbundle By Name(w529) -> ("Data"=w521:T1)
          n194 = call-poly "CoreLib.byte array 2 data.vi"("byteArray"=w521) -> ("i16"=w520:i16, "error out"=w519:errorcluster)  [unwired: 16 in, 1 out]
          n195 = Not Equal To 0?(x=w520) -> (x != 0?=w517:bool)
          n196 = case shown="No Error" w519 {
            tunnel: [w545 w549] -> w526
            tunnel: w532 -> [w541 w549]
            tunnel: w531 -> [w540 w548]
            tunnel: [w544 w547] -> w525
            tunnel: w523 -> [_ w546]
            tunnel: w517 -> [w543 _]
            tunnel: w518 -> [w542 _]
            frame No Error {
              n197 = call "AFG3352X.get i attribute.vi"("i ref in"=w541, "error in (no error)"=w540) -> ("i ref out"=w538:refnum<vi>, "i attribute"=w537:T4, "error out"=w539:errorcluster)  [unwired: 15 in]
              n198 = Unbundle By Name(w537) -> ("DefaultChannel"=w536:i32)
              n199 = call "AFG3352X.enable output.vi"("i ref in"=w538, "Channel (1: 1)"=w536, "outputEnable"=w543, "ms timeout (10000)"=w542, "error in (no error)"=w539) -> ("i ref out"=w545:refnum<vi>, "error out"=w544:errorcluster)  [unwired: 12 in, 1 out]
            }
            frame Error {
              n200 = call "CoreLib.set data type mismatch.vi"("error in (no error)"=w548, "error source"=w546) -> ("error out"=w547:errorcluster)  [unwired: 17 in]
            }
          }
          n201 = call "BaseProcess.set event status.vi"("i ref in"=w526, "EventStatus"=w523, "error in (no error)"=w525) -> ("i ref out"=w522:refnum<vi>, "error out"=w524:errorcluster)  [unwired: 14 in, 1 out]
          n202 = case shown="Error" w524 {
            selector: w524 -> [_ w535]
            tunnel: [_ w534] -> w527
            frame No Error {
            }
            frame Error {
              n203 = Unbundle By Name(w535) -> ("source"=w533:string)
              n204 = call-poly "CoreLib.data 2 byte array.vi"("string"=w533) -> ("byteArray out"=w534:T1)  [unwired: 18 in]
            }
          }
          n205 = Unbundle By Name(w524) -> ("code"=w530:i32)
          n206 = Bundle By Name(cluster=w529, "Data"=w527, "Error #"=w530) -> (w528:T2)
        }
        frame "SetChannelOutputEnabled" {
          n207 = Unbundle By Name(w565) -> ("Data"=w553:T1)
          n208 = call-poly "CoreLib.byte array 2 data.vi"("byteArray"=w553) -> ("byteArray out"=w552:T1, "i32"=w550:i32, "error out"=w551:errorcluster)  [unwired: 16 in]
          n209 = call-poly "CoreLib.byte array 2 data.vi"("byteArray"=w552, "error in (no error)"=w551) -> ("i16"=w557:i16, "error out"=w556:errorcluster)  [unwired: 15 in, 1 out]
          n210 = Not Equal To 0?(x=w557) -> (x != 0?=w554:bool)
          n211 = case shown="No Error" w556 {
            tunnel: [w578 w582] -> w562
            tunnel: w568 -> [w573 w582]
            tunnel: w567 -> [w574 w581]
            tunnel: [w577 w580] -> w561
            tunnel: w559 -> [_ w579]
            tunnel: w554 -> [w576 _]
            tunnel: w555 -> [w575 _]
            tunnel: w550 -> [w572 _]
            frame No Error {
              n212 = call "AFG3352X.enable output.vi"("i ref in"=w573, "Channel (1: 1)"=w572, "outputEnable"=w576, "ms timeout (10000)"=w575, "error in (no error)"=w574) -> ("i ref out"=w578:refnum<vi>, "error out"=w577:errorcluster)  [unwired: 12 in, 1 out]
            }
            frame Error {
              n213 = call "CoreLib.set data type mismatch.vi"("error in (no error)"=w581, "error source"=w579) -> ("error out"=w580:errorcluster)  [unwired: 17 in]
            }
          }
          n214 = call "BaseProcess.set event status.vi"("i ref in"=w562, "EventStatus"=w559, "error in (no error)"=w561) -> ("i ref out"=w558:refnum<vi>, "error out"=w560:errorcluster)  [unwired: 14 in, 1 out]
          n215 = case shown="Error" w560 {
            selector: w560 -> [_ w571]
            tunnel: [_ w570] -> w563
            frame No Error {
            }
            frame Error {
              n216 = Unbundle By Name(w571) -> ("source"=w569:string)
              n217 = call-poly "CoreLib.data 2 byte array.vi"("string"=w569) -> ("byteArray out"=w570:T1)  [unwired: 18 in]
            }
          }
          n218 = Unbundle By Name(w560) -> ("code"=w566:i32)
          n219 = Bundle By Name(cluster=w565, "Data"=w563, "Error #"=w566) -> (w564:T2)
        }
        frame "SetTrigger" {
          n220 = Unbundle By Name(w594) -> ("Data"=w586:T1)
          n221 = call-poly "CoreLib.byte array 2 data.vi"("byteArray"=w586) -> ("[i16]"=w583:i16[], "error out"=w585:errorcluster)  [unwired: 16 in, 1 out]
          n222 = case shown="No Error" w585 {
            tunnel: [w605 w610] -> w591
            tunnel: w597 -> [w606 w610]
            tunnel: w596 -> [w603 w609]
            tunnel: [w604 w608] -> w590
            tunnel: w588 -> [_ w607]
            tunnel: w583 -> [w602 _]
            tunnel: w584 -> [w601 _]
            frame No Error {
              n223 = call "AFG3352X.set trigger.vi"("i ref in"=w606, "triggerParameters"=w602, "ms timeout (10000)"=w601, "error in (no error)"=w603) -> ("i ref out"=w605:refnum<vi>, "error out"=w604:errorcluster)  [unwired: 13 in, 1 out]
            }
            frame Error {
              n224 = call "CoreLib.set data type mismatch.vi"("error in (no error)"=w609, "error source"=w607) -> ("error out"=w608:errorcluster)  [unwired: 17 in]
            }
          }
          n225 = call "BaseProcess.set event status.vi"("i ref in"=w591, "EventStatus"=w588, "error in (no error)"=w590) -> ("i ref out"=w587:refnum<vi>, "error out"=w589:errorcluster)  [unwired: 14 in, 1 out]
          n226 = case shown="Error" w589 {
            selector: w589 -> [_ w600]
            tunnel: [_ w599] -> w592
            frame No Error {
            }
            frame Error {
              n227 = Unbundle By Name(w600) -> ("source"=w598:string)
              n228 = call-poly "CoreLib.data 2 byte array.vi"("string"=w598) -> ("byteArray out"=w599:T1)  [unwired: 18 in]
            }
          }
          n229 = Unbundle By Name(w589) -> ("code"=w595:i32)
          n230 = Bundle By Name(cluster=w594, "Data"=w592, "Error #"=w595) -> (w593:T2)
        }
        frame "Configure" {
          n231 = Unbundle By Name(w623) -> ("Data"=w615:T1)
          n232 = call-poly "CoreLib.byte array 2 data.vi"("byteArray"=w615) -> ("string"=w612:string, "error out"=w614:errorcluster)  [unwired: 16 in, 1 out]
          n233 = call "CoreLib.stringToStringArray.vi"("String"=w612) -> ("Array"=w611:string[])
          n234 = case shown="No Error" w614 {
            tunnel: [w634 w639] -> w620
            tunnel: w626 -> [w635 w639]
            tunnel: w625 -> [w632 w638]
            tunnel: [w633 w637] -> w619
            tunnel: w617 -> [_ w636]
            tunnel: w611 -> [w631 _]
            tunnel: w613 -> [w630 _]
            frame No Error {
              n235 = call "AFG3352X.configure.vi"("i ref in"=w635, "configureData"=w631, "ms timeout (10000)"=w630, "error in (no error)"=w632) -> ("i ref out"=w634:refnum<vi>, "error out"=w633:errorcluster)  [unwired: 13 in, 1 out]
            }
            frame Error {
              n236 = call "CoreLib.set data type mismatch.vi"("error in (no error)"=w638, "error source"=w636) -> ("error out"=w637:errorcluster)  [unwired: 17 in]
            }
          }
          n237 = call "BaseProcess.set event status.vi"("i ref in"=w620, "EventStatus"=w617, "error in (no error)"=w619) -> ("i ref out"=w616:refnum<vi>, "error out"=w618:errorcluster)  [unwired: 14 in, 1 out]
          n238 = case shown="Error" w618 {
            selector: w618 -> [_ w629]
            tunnel: [_ w628] -> w621
            frame No Error {
            }
            frame Error {
              n239 = Unbundle By Name(w629) -> ("source"=w627:string)
              n240 = call-poly "CoreLib.data 2 byte array.vi"("string"=w627) -> ("byteArray out"=w628:T1)  [unwired: 18 in]
            }
          }
          n241 = Unbundle By Name(w618) -> ("code"=w624:i32)
          n242 = Bundle By Name(cluster=w623, "Data"=w621, "Error #"=w624) -> (w622:T2)
        }
        frame "UseAM" {
          n243 = call "AFG3352X.use external amplitude modulation.vi"("i ref in"=w651, "ms timeout (10000)"=w640, "error in (no error)"=w650) -> ("i ref out"=w645:refnum<vi>, "error out"=w644:errorcluster)  [unwired: 14 in, 1 out]
          n244 = call "BaseProcess.set event status.vi"("i ref in"=w645, "EventStatus"=w642, "error in (no error)"=w644) -> ("i ref out"=w641:refnum<vi>, "error out"=w643:errorcluster)  [unwired: 14 in, 1 out]
          n245 = case shown="Error" w643 {
            selector: w643 -> [_ w654]
            tunnel: [_ w653] -> w646
            frame No Error {
            }
            frame Error {
              n246 = Unbundle By Name(w654) -> ("source"=w652:string)
              n247 = call-poly "CoreLib.data 2 byte array.vi"("string"=w652) -> ("byteArray out"=w653:T1)  [unwired: 18 in]
            }
          }
          n248 = Unbundle By Name(w643) -> ("code"=w649:i32)
          n249 = Bundle By Name(cluster=w648, "Data"=w646, "Error #"=w649) -> (w647:T2)
        }
        frame "Initialize" {
          n250 = Unbundle By Name(w661) -> ("Data"=w662:T1)
          n251 = call-poly "CoreLib.byte array 2 data.vi"("byteArray"=w662) -> ("byteArray out"=w660:T1, "i16"=w656:i16, "error out"=w659:errorcluster)  [unwired: 16 in]
          n252 = call-poly "CoreLib.byte array 2 data.vi"("byteArray"=w660, "error in (no error)"=w659) -> ("i16"=w655:i16, "error out"=w658:errorcluster)  [unwired: 15 in, 1 out]
          n253 = case shown="No Error" w658 {
            tunnel: [w686 w690] -> w671
            tunnel: [w685 w688] -> w670
            tunnel: w667 -> [w684 _]
            tunnel: w666 -> [w682 w689]
            tunnel: w665 -> [w681 w690]
            tunnel: [w679 _] -> w664
            tunnel: w657 -> [_ w687]
            tunnel: w656 -> [w678 _]
            tunnel: w655 -> [w676 _]
            frame No Error {
              n254 = Not Equal To 0?(x=w678) -> (x != 0?=w677:bool)
              n255 = Not Equal To 0?(x=w676) -> (x != 0?=w675:bool)
              n256 = call "AFG3352X.close.vi"("i ref in"=w681, "ms timeout (10000)"=w684, "error in (no error)"=w682) -> ("i ref out"=w680:refnum<vi>, "error out"=w683:errorcluster)  [unwired: 14 in, 1 out]
              n257 = call "AFG3352X.initialize.vi"("i ref in"=w680, "queryID"=w677, "resetDevice"=w675, "ms timeout (10000)"=w684, "error in (no error)"=w683) -> ("i ref out"=w686:refnum<vi>, "deviceID"=w679:string, "error out"=w685:errorcluster)  [unwired: 11 in, 1 out]
            }
            frame Error {
              n258 = call "CoreLib.set data type mismatch.vi"("error in (no error)"=w689, "error source"=w687) -> ("error out"=w688:errorcluster)  [unwired: 17 in]
            }
          }
          n259 = call "BaseProcess.set event status.vi"("i ref in"=w671, "EventStatus"=w657, "error in (no error)"=w670) -> ("i ref out"=w668:refnum<vi>, "error out"=w669:errorcluster)  [unwired: 14 in, 1 out]
          n260 = case shown="No Error" w669 {
            selector: w669 -> [_ w695]
            tunnel: [w692 w694] -> w672
            tunnel: w664 -> [w691 _]
            frame No Error {
              n261 = call-poly "CoreLib.data 2 byte array.vi"("string"=w691) -> ("byteArray out"=w692:T1)  [unwired: 18 in]
            }
            frame Error {
              n262 = Unbundle By Name(w695) -> ("source"=w693:string)
              n263 = call-poly "CoreLib.data 2 byte array.vi"("string"=w693) -> ("byteArray out"=w694:T1)  [unwired: 18 in]
            }
          }
          n264 = Unbundle By Name(w669) -> ("code"=w674:i32)
          n265 = Bundle By Name(cluster=w661, "Data"=w672, "Error #"=w674, "Data Descriptor"=T3 "C:N") -> (w673:T2)
        }
        frame "Close" {
          n266 = call "AFG3352X.close.vi"("i ref in"=w698, "ms timeout (10000)"=w700, "error in (no error)"=w699) -> ("i ref out"=w697:refnum<vi>, "error out"=w696:errorcluster)  [unwired: 14 in, 1 out]
          n267 = call "BaseProcess.set event status.vi"("i ref in"=w697, "EventStatus"=w702, "error in (no error)"=w696) -> ("i ref out"=w701:refnum<vi>, "error out"=w703:errorcluster)  [unwired: 14 in, 1 out]
          n268 = case shown="Error" w703 {
            selector: w703 -> [_ w710]
            tunnel: [_ w709] -> w704
            frame No Error {
            }
            frame Error {
              n269 = Unbundle By Name(w710) -> ("source"=w708:string)
              n270 = call-poly "CoreLib.data 2 byte array.vi"("string"=w708) -> ("byteArray out"=w709:T1)  [unwired: 18 in]
            }
          }
          n271 = Unbundle By Name(w703) -> ("code"=w707:i32)
          n272 = Bundle By Name(cluster=w706, "Data"=w704, "Error #"=w707) -> (w705:T2)
        }
        frame "Reset" {
          n273 = call "BaseProcess.set event status.vi"("i ref in"=w712, "EventStatus"=w714, "error in (no error)"=w711) -> ("i ref out"=w713:refnum<vi>, "error out"=w715:errorcluster)  [unwired: 14 in, 1 out]
          n274 = case shown="Error" w715 {
            selector: w715 -> [_ w722]
            tunnel: [_ w721] -> w716
            frame No Error {
            }
            frame Error {
              n275 = Unbundle By Name(w722) -> ("source"=w720:string)
              n276 = call-poly "CoreLib.data 2 byte array.vi"("string"=w720) -> ("byteArray out"=w721:T1)  [unwired: 18 in]
            }
          }
          n277 = Unbundle By Name(w715) -> ("code"=w719:i32)
          n278 = Bundle By Name(cluster=w718, "Data"=w716, "Error #"=w719) -> (w717:T2)
        }
      }
    }
    frame Error {
    }
  }
  "answer cluster" <- w8
  "i ref out" <- w4
  "error out" <- w3
